vi "PLC Struct Byte Stream to G Object 2.vi"(7 "Type Name":string, 8 "error in (no error)":errorcluster, 9 "[Sub-Item Type Information]":T1[](array[typedef]), 10 "Byte Stream":u8[](array[numeric]), 11 "TwinCAT ADS in":refnum<class "TwinCAT ADS.lvclass">) -> (0 "error out":errorcluster, 2 "Value":variant, 3 "TwinCAT ADS out":refnum<class "TwinCAT ADS.lvclass">)   [LabVIEW 2018]
uses:
  TwinCAT ADS.lvclass
  Controls/PLC Type.ctl
  Controls/PLC Sub-Item Type Descriptor.ctl
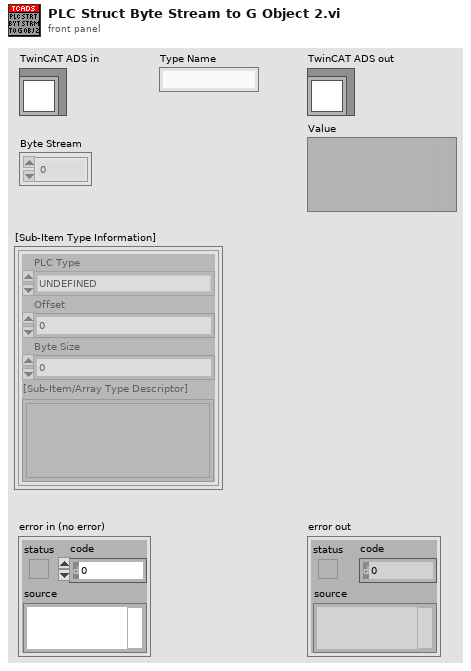
[diagram p1: front panel]
types:
  T1 = typedef "TwinCAT ADS.lvclass/PLC Sub-Item Type Descriptor.ctl" = cluster{"PLC Type":T2, "Offset":i32, "Byte Size":i32, "[Sub-Item/Array Type Descriptor]":variant[]}
  T2 = typedef "TwinCAT ADS.lvclass/PLC Type.ctl" = enum16{"UNDEFINED", "INT", "DINT", "REAL", "LREAL", "SINT", "BYTE", "UINT", "UDINT", "LINT", "ULINT", "STRING", "WSTRING", "BOOL", "TIME", "LTIME", "DATE", "DT", "TOD", "ARRAY", "JAGGED ARRAY", "STRUCT", "FUNCTION BLOCK", "POINTER", "USER DEFINED"}
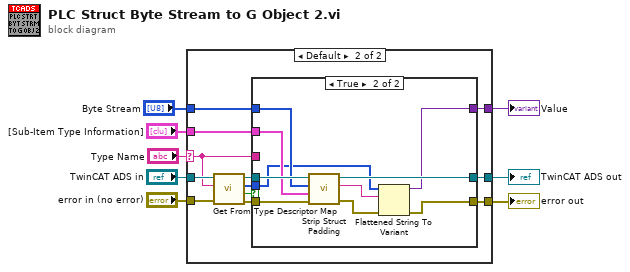
[diagram p0: block diagram]
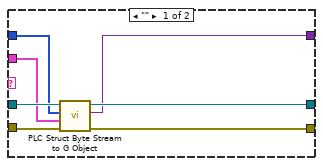
[diagram p2: hidden frame]
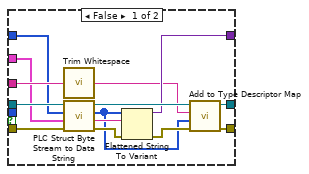
[diagram p3: hidden frame]
diagram:
  n1 = case shown="Default" "Type Name" {
    selector: "Type Name" -> [_ w16]
    tunnel: "TwinCAT ADS in" -> [w15 w26]
    tunnel: "Byte Stream" -> [w10 w20]
    tunnel: "error in (no error)" -> [w14 w25]
    tunnel: "[Sub-Item Type Information]" -> [w13 w21]
    tunnel: [w11 w19] -> w4
    tunnel: [w12 w18] -> w3
    tunnel: [w9 w17] -> w2
    frame "" {
      n2 = call "PLC Struct Byte Stream to G Object.vi"("error in (no error)"=w14, "[Sub-Item Type Information]"=w13, "Byte Stream"=w10, "TwinCAT ADS in"=w15) -> ("error out"=w12:errorcluster, "Value"=w9:variant, "TwinCAT ADS out"=w11:refnum<class "TwinCAT ADS.lvclass">)  [unwired: 5 in]
    }
    frame Default {
      n3 = call "Get From Type Descriptor Map.vi"("error in (no error)"=w25, "Type Name"=w16, "TwinCAT ADS in"=w26) -> ("error out"=w24:errorcluster, "Found?"=w23:bool, "Type Descriptor"=w22:i16[], "TwinCAT ADS out"=w27:refnum<class "TwinCAT ADS.lvclass">)  [unwired: 5 in]
      n4 = case shown="True" w23 {
        tunnel: w24 -> [w34 w49]
        tunnel: w22 -> [_ w42]
        tunnel: w27 -> [w35 w51]
        tunnel: w21 -> [w33 w44]
        tunnel: w20 -> [w32 w43]
        tunnel: [w39 w50] -> w19
        tunnel: [w40 w46] -> w18
        tunnel: [w37 w45] -> w17
        tunnel: w16 -> [w36 _]
        frame False {
          n5 = call <vilib>:"Trim Whitespace.vi"("string"=w36) -> ("trimmed string"=w28:string)  [unwired: 1 in]
          n6 = call "PLC Struct Byte Stream to Data String.vi"("error in (no error)"=w34, "[Sub-Item Type Information]"=w33, "Byte Stream"=w32, "TwinCAT ADS in"=w35) -> ("error out"=w31:errorcluster, "Data String"=w30:string, "Type Descriptor"=w29:i16[], "TwinCAT ADS out"=w41:refnum<class "TwinCAT ADS.lvclass">)  [unwired: 4 in]
          n7 = Flattened String To Variant(4:w31, 6:w30, 7:w29) -> (0:w38:errorcluster, 3:w37:variant)
          n8 = call "Add to Type Descriptor Map.vi"("error in (no error)"=w38, "Type Descriptor"=w29, "Type Name"=w28, "TwinCAT ADS in"=w41) -> ("error out"=w40:errorcluster, "TwinCAT ADS out"=w39:refnum<class "TwinCAT ADS.lvclass">)  [unwired: 5 in, 1 out]
        }
        frame True {
          n9 = call "Strip Struct Padding.vi"("error in (no error)"=w49, "[Sub-Item Type Information]"=w44, "Byte Stream in"=w43, "TwinCAT ADS in"=w51) -> ("error out"=w48:errorcluster, "Data String"=w47:string, "TwinCAT ADS out"=w50:refnum<class "TwinCAT ADS.lvclass">)  [unwired: 5 in]
          n10 = Flattened String To Variant(4:w48, 6:w47, 7:w42) -> (0:w46:errorcluster, 3:w45:variant)
        }
      }
    }
  }
  "error out" <- w3
  "TwinCAT ADS out" <- w4
  "Value" <- w2
